vi "SLL DE Compare Enum and MAX Channel.vi"(8 "error in (no error)":errorcluster, 10 "Strings []":string[](array[string]), 11 "Channels In":refnum<k21>[](array[refnum])) -> (0 "error out":errorcluster, 2 "Pass?":bool, 3 "Channels Out":refnum<k21>[](array[refnum]))   [LabVIEW 2013]
doc: "This VI will check and seperate all Analog Inputs listed in enum form global Channel list\n\nCreated by Yogesh Redemptor, \nCopyright © 2008, Soliton Technologies.\nAll rights reserved."
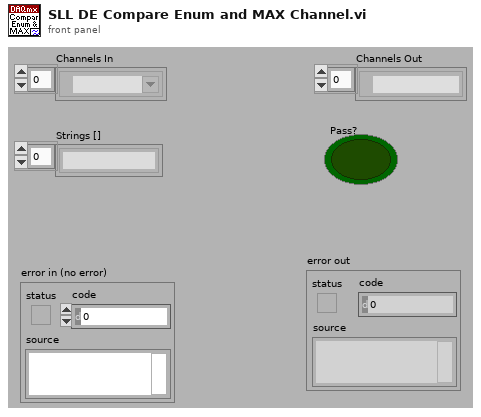
[diagram p1: front panel]
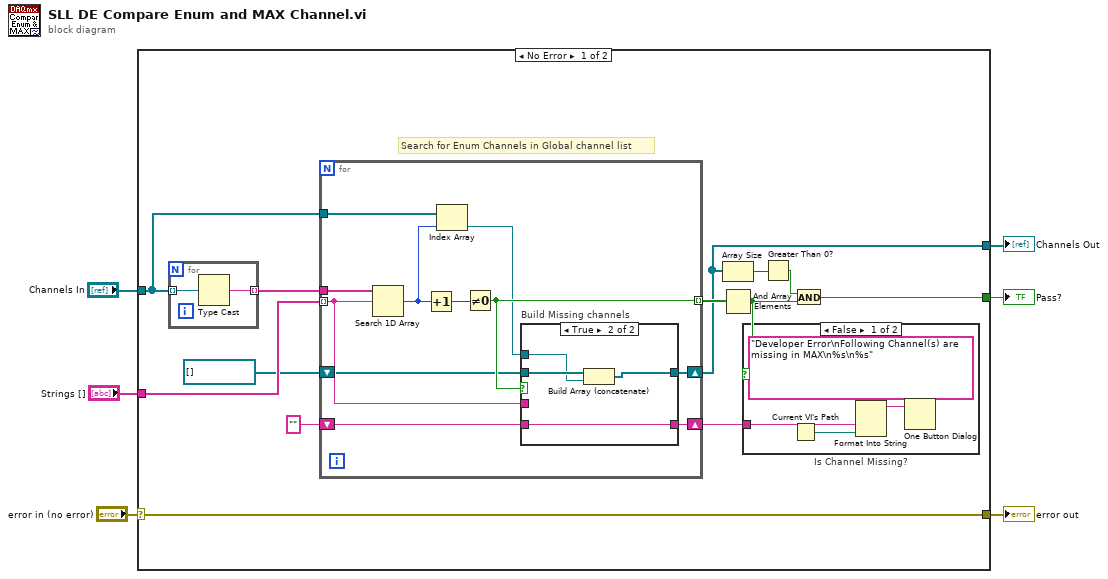
[diagram p0: block diagram]
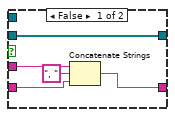
[diagram p3: hidden frame]
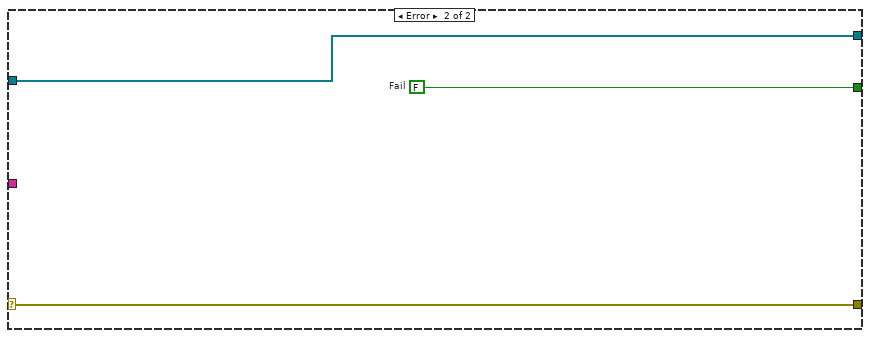
[diagram p4: hidden frame]
diagram:
  n1 = case shown="No Error" "error in (no error)" {
    selector: "error in (no error)" -> [w9 w48]
    tunnel: [w9 w48] -> w5
    tunnel: "Channels In" -> [w17 w47]
    tunnel: [w15 w46] -> w3
    tunnel: [w7 w47] -> w2
    tunnel: "Strings []" -> [w10 _]
    frame No Error {
      # "Search for Enum Channels in Global channel list"
      n2 = for {
        tunnel: w17 -> [w45] mode=indexing
        tunnel: [w44] -> w19 mode=indexing
        n3 = Type Cast(x=w45) -> (*(type *) &x=w44:string)  [unwired: 1 out]
      }
      n4 = for {
        tunnel: w19 -> [w34]
        tunnel: w10 -> [w29] mode=indexing
        tunnel: [w30] -> w18 mode=indexing
        tunnel: w17 -> [w32]
        shift-right: [w27] -> w12
        shift-left: "" -> [w28]
        shift-right: [w25] -> w7
        shift-left: refnum<k21>[] [] -> [w24]
        n5 = Search 1D Array(1D array=w34, element=w29) -> (index of element=w31:i32)  [unwired: 1 out]
        n6 = Increment(x=w31) -> (x+1=w33:i32)
        n7 = Index Array(array=w32, index=w31) -> (element=w26:refnum<k21>)
        n8 = Not Equal To 0?(x=w33) -> (x != 0?=w30:bool)
        n9 = case "Build Missing channels" shown="True" w30 {
          tunnel: w29 -> [w39 _]
          tunnel: [w38 w43] -> w27
          tunnel: w28 -> [w36 w43]
          tunnel: w26 -> [_ w41]
          tunnel: [w35 w40] -> w25
          tunnel: w24 -> [w35 w42]
          frame False {
            n10 = Concatenate Strings(w39, ", " ("string"), w36) -> (w38:string)
          }
          frame True {
            n11 = Build Array (concatenate)(w42, w41) -> (w40:refnum<k21>[])
          }
        }
      }
      n12 = Array Size(array=w7) -> (size(s)=w16:i32)
      n13 = And Array Elements(Boolean array=w18) -> (logical AND=w11:bool)
      n14 = case "Is Channel Missing?" shown="False" w11 {
        tunnel: w12 -> [w20 _]
        frame False {
          n15 = Current VI's Path() -> (path=w21:path)
          n16 = Format Into String(format string="Developer Error\nFollowing Channel(s) are missing in MAX\n%s\n%s" ("message"), w20, w21) -> (resulting string=w22:string)  [unwired: 2 in, 1 out]
          n17 = One Button Dialog(message=w22) -> ()  [unwired: 1 in, 1 out]
        }
        frame True {
        }
      }
      n18 = Greater Than 0?(x=w16) -> (x > 0?=w14:bool)
      n19 = And(x=w14, y=w11) -> (x .and. y?=w15:bool)
    }
    frame Error {
      w46 = FALSE  # Fail
    }
  }
  "error out" <- w5
  "Pass?" <- w3
  "Channels Out" <- w2
